vi "export Complex Data 1D.vi"(4 "error in (no error)":errorcluster, 5 "Export File":path, 6 "Data 2D Export Format Selection":T1, 7 "Data in":refnum<class "Data.lvclass">) -> (0 "error out":errorcluster, 3 "Data out":refnum<class "Data.lvclass">)   [LabVIEW 2017]
uses:
  C:/Program Files/Thorlabs/SpectralRadar/LabVIEW/2012/user.lib/SpectralRadar.llb/Data.lvclass
  C:/Program Files/Thorlabs/SpectralRadar/LabVIEW/2012/user.lib/SpectralRadar.llb/Data 2D Export Format Selection.ctl
  SpectralRadar.dll
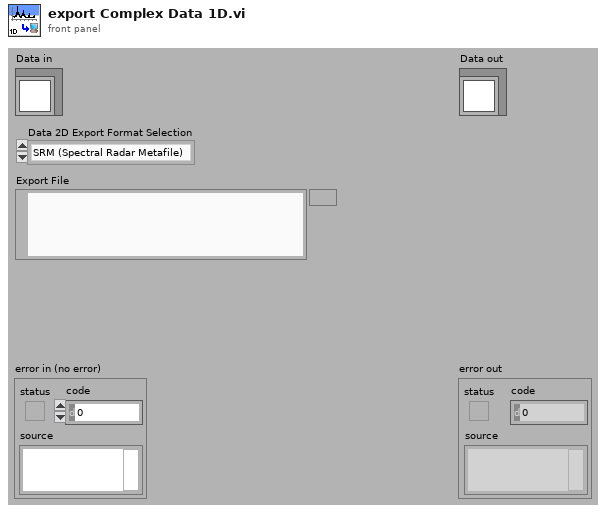
[diagram p1: front panel]
types:
  T1 = typedef "Data.lvclass/Data 2D Export Format Selection.ctl" = enum16{"SRM (Spectral Radar Metafile)", "RAW", "TXT", "CSV", "TXT Table"}
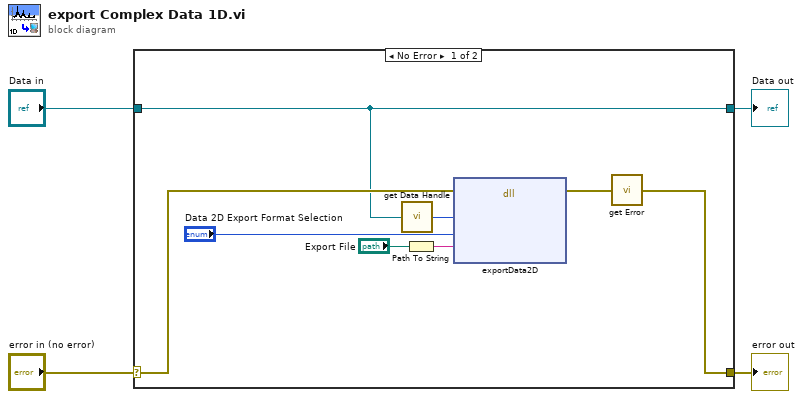
[diagram p0: block diagram]
diagram:
  n1 = case shown="No Error" "error in (no error)" {
    selector: "error in (no error)" -> [w12 w14]
    tunnel: [w5 w14] -> w3
    tunnel: [w10 w13] -> w1
    tunnel: "Data in" -> [w10 w13]
    frame No Error {
      n2 = call "get Data Handle.vi"("Data"=w10) -> ("Handle"=w9:u64)
      n3 = Path To String(path="Export File") -> (string=w8:string)
      n4 = dll-call lib="SpectralRadar.dll" fn="exportData2D"(error in=w12, "Data Handle"=w9, "Export Format"="Data 2D Export Format Selection", "File Name"=w8) -> (error out=w6:errorcluster)  [unwired: 6 in, 1 out]
      n5 = call "get Error.vi"("error in (no error)"=w6) -> ("error out"=w5:errorcluster)
    }
    frame Error {
    }
  }
  "error out" <- w3
  "Data out" <- w1
